vi "Get Invalid Group Scalar Channels.vi"(7 "invalid group scalars in":T2[](array[typedef]) {"Data Type" format="%.0x"}, 8 "error in":errorcluster, 9 "new bitfile scalar channels":T2 {"Data Type" format="%.0x"}, 10 "old bitfile scalar channels":T2 {"Data Type" format="%.0x"}, 11 "item ref in":T1 format="%.0x") -> (0 "error out":errorcluster, 2 "invalid group scalars out":T2[](array[typedef]) {"Data Type" format="%.0x"}, 3 "item ref out":T1 format="%.0x")   [LabVIEW 2018, in "FPGA Addon System Explorer.lvlib"]
uses:
  FPGA Addon System Explorer.lvlib
  Addon Shared/Types/Register Information.ctl
  Addon Shared/Types/Data Type.ctl
  <vilib>/NI Veristand/Custom Device API/Custom Device Item Ref.ctl
  Addon Shared/FPGA Addon Shared.lvlib
  <vilib>/NI Veristand/Custom Device API/Custom Device API.lvlib
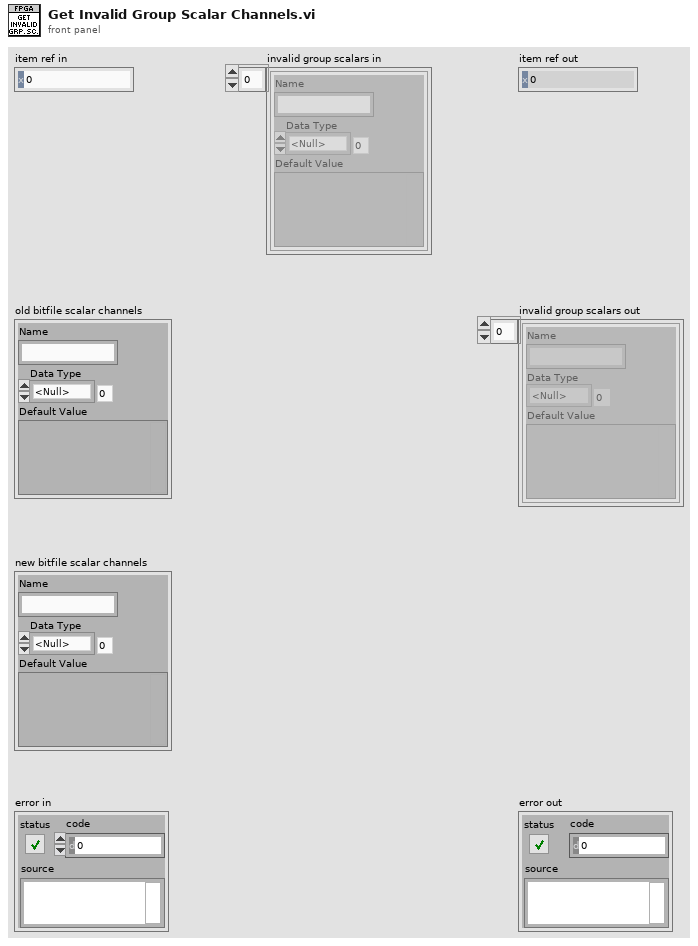
[diagram p1: front panel]
types:
  T1 = typedef "Custom Device API.lvlib/Custom Device Item Ref.ctl" = u64
  T2 = typedef "FPGA Addon Shared.lvlib/Register Information.ctl" = cluster{"Name":string, "Data Type":T3, "Default Value":variant}
  T3 = typedef "FPGA Addon Shared.lvlib/Data Type.ctl" = enum8{"<Null>", "I8", "I16", "I32", "I64", "U8", "U16", "U32", "U64", "SGL", "Boolean", "Analog PWM In Settings", "Analog PWM In", "Digital PWM In Settings", "Digital PWM In", "Digital PWM Out", "Sine Out", "FXP+/-24.5", "FXP+/-16.5", "FXP+/-32.8", "FXP+/-64.32", "FXP+/-16.7", "FXP+/-20.5", "FXP+/-27.5", "FXP+/-32.16", "FXP+16.3", "FXP+18.3", "Digital Static In", "Digital Static Out", "Digital Static In Settings", "Digital WSS Out", "Quad Encoder Settings", "Quad Encoder In", "Group"}
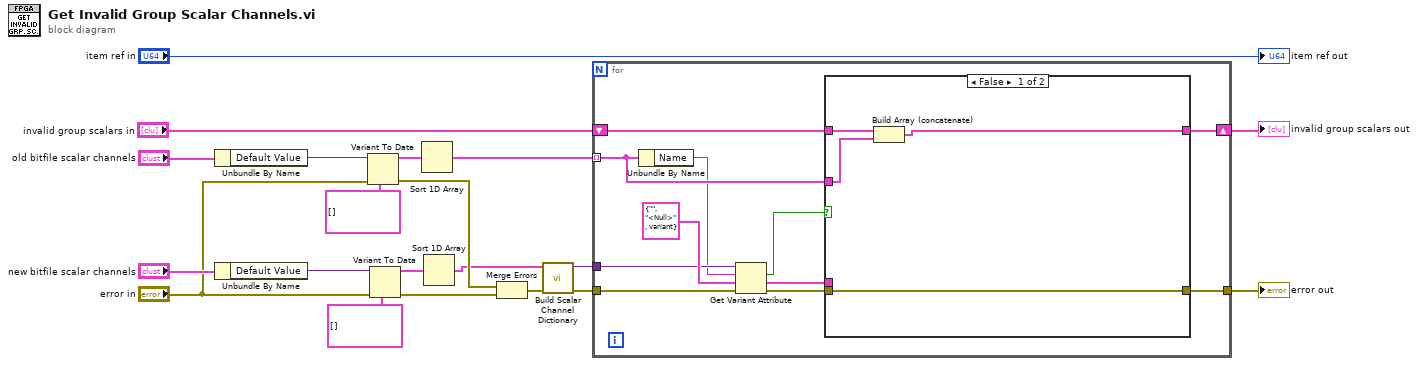
[diagram p0: block diagram]
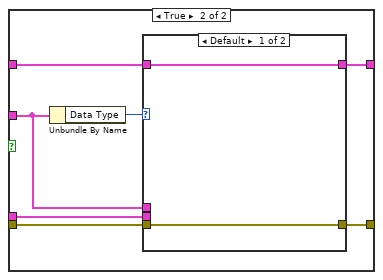
[diagram p2: hidden frame]
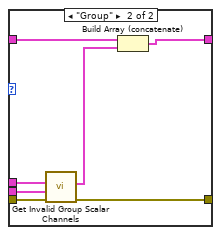
[diagram p3: hidden frame]
diagram:
  n1 = Unbundle By Name("old bitfile scalar channels") -> ("Default Value"=w16:variant)
  n2 = Unbundle By Name("new bitfile scalar channels") -> ("Default Value"=w13:variant)
  n3 = Variant To Data(error in="error in", type=T2[] [], Variant=w16) -> (data=w17:T2[], error out=w12:errorcluster)
  n4 = Variant To Data(error in="error in", type=T2[] [], Variant=w13) -> (data=w18:T2[], error out=w11:errorcluster)
  n5 = Sort 1D Array(array=w17) -> (sorted array=w8:T2[])
  n6 = Sort 1D Array(array=w18) -> (sorted array=w5:T2[])
  n7 = Merge Errors(w12, w11) -> (w6:errorcluster)
  n8 = call "Build Scalar Channel Dictionary.vi"("error in (no error)"=w6, "new bitfile scalar channels"=w5) -> ("error out"=w4:errorcluster, "scalar channels dictionary"=w3:variant)  [unwired: 8 in]
  n9 = for {
    tunnel: w4 -> [w28]
    tunnel: w8 -> [w24] mode=indexing
    tunnel: w3 -> [w26]
    tunnel: [w22] -> w7
    shift-right: [w30] -> w1
    shift-left: "invalid group scalars in" -> [w31]
    n10 = Unbundle By Name(w24) -> ("Name"=w21:string)
    n11 = Get Variant Attribute(Variant=w26, name=w21, default value (empty Variant)=T2 {"Name"="", "Data Type"=enum."<Null>", "Default Value"=variant}, error in=w28) -> (found=w25:bool, value=w23:T2, error out=w27:errorcluster)  [unwired: 1 out]
    n12 = case shown="False" w25 {
      tunnel: w31 -> [w35 w42]
      tunnel: [w32 w41] -> w30
      tunnel: w27 -> [w34 w37]
      tunnel: w24 -> [w33 w39]
      tunnel: w23 -> [_ w38]
      tunnel: [w34 w36] -> w22
      frame False {
        n13 = Build Array (concatenate)(w35, w33) -> (w32:T2[])
      }
      frame True {
        n14 = Unbundle By Name(w39) -> ("Data Type"=w40:T3)
        n15 = case shown="Default" w40 {
          tunnel: w42 -> [w44 w46]
          tunnel: [w44 w45] -> w41
          tunnel: w39 -> [_ w48]
          tunnel: w38 -> [_ w49]
          tunnel: w37 -> [w43 w51]
          tunnel: [w43 w50] -> w36
          frame Default {
          }
          frame "Group" {
            n16 = call "Get Invalid Group Scalar Channels.vi"("error in"=w51, "new bitfile scalar channels"=w49, "old bitfile scalar channels"=w48) -> ("error out"=w50:errorcluster, "invalid group scalars out"=w47:T2[])  [unwired: 6 in, 1 out]
            n17 = Build Array (concatenate)(w46, w47) -> (w45:T2[])
          }
        }
      }
    }
  }
  "error out" <- w7
  "invalid group scalars out" <- w1
  "item ref out" <- "item ref in"
